vi "Send Schedule to Local Searcher.vi"(8 "error in (no error)":errorcluster, 9 "Schedule":u16[](array[numeric]), 10 "queue in":refnum<queue>, 11 "OSSP_Problem in":refnum<class "OSSP_Problem.lvclass">) -> (0 "error out":errorcluster, 3 "OSSP_Problem out":refnum<class "OSSP_Problem.lvclass">)   [LabVIEW 2013]
uses:
  Classes/OSSP_Problem.lvclass
  Required Data for LSA.ctl
  Classes/OSSP_Problem.lvclass/OSSP_Problem.ctl
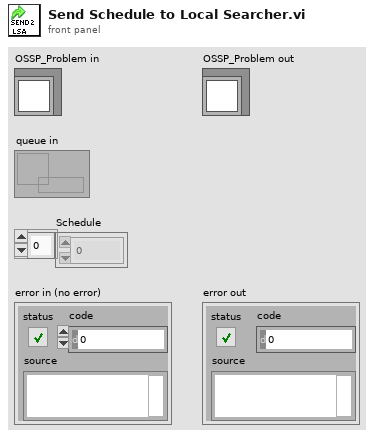
[diagram p1: front panel]
types:
  T1 = typedef "Required Data for LSA.ctl" = cluster{"Number of Machines":i32, "Number of Jobs":i32, "Due Dates":u16[], "Processing Times":u16[][], "Schedule":u16[]}
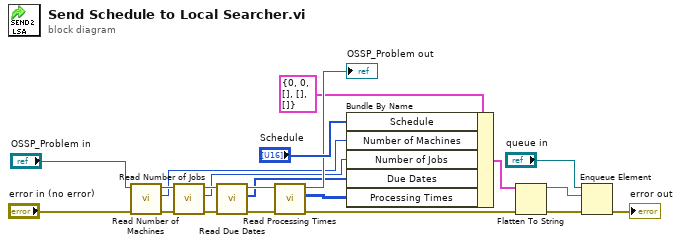
[diagram p0: block diagram]
diagram:
  n1 = call "Read Number of Machines.vi"("error in (no error)"="error in (no error)", "OSSP_Problem in"="OSSP_Problem in") -> ("error out"=w15:errorcluster, "Number of Machines"=w9:i32, "OSSP_Problem out"=w12:refnum<class "OSSP_Problem.lvclass">)  [unwired: 7 in]
  n2 = call "Read Number of Jobs.vi"("error in (no error)"=w15, "OSSP_Problem in"=w12) -> ("error out"=w14:errorcluster, "Number of Jobs"=w8:i32, "OSSP_Problem out"=w11:refnum<class "OSSP_Problem.lvclass">)  [unwired: 7 in]
  n3 = call "Read Due Dates.vi"("error in (no error)"=w14, "OSSP_Problem in"=w11) -> ("error out"=w13:errorcluster, "Due Dates"=w6:u16[], "OSSP_Problem out"=w10:refnum<class "OSSP_Problem.lvclass">)  [unwired: 7 in]
  n4 = call "Read Processing Times.vi"("error in (no error)"=w13, "OSSP_Problem in"=w10) -> ("error out"=w2:errorcluster, "Processing Times"=w5:u16[][], "OSSP_Problem out"=→"OSSP_Problem out":refnum<class "OSSP_Problem.lvclass">)  [unwired: 7 in]
  n5 = Bundle By Name(cluster=T1 {"Number of Machines"=0, "Number of Jobs"=0, "Due Dates"=[], "Processing Times"=[], "Schedule"=[]}, "Schedule"="Schedule", "Number of Machines"=w9, "Number of Jobs"=w8, "Due Dates"=w6, "Processing Times"=w5) -> (w4:T1)
  n6 = Flatten To String(anything=w4, error in (no error)=w2) -> (data string=w3:string, error out=w1:errorcluster)  [unwired: 2 in, 1 out]
  n7 = Enqueue Element(queue="queue in", element=w3, error in (no error)=w1) -> (error out=→"error out":errorcluster)  [unwired: 1 in, 2 out]
